vi "MT Generate MSK System Parameters.vi"(0 "samples per symbol (16)":i32=16, 5 "differential encoding enable":enum16{"disable", "enable"}(ring)=enum."enable", 11 "error in (no error)":errorcluster) -> (6 "MSK system parameters":T1, 8 "bits per symbol":i32, 15 "error out":errorcluster)   [LabVIEW 2020, in "niDMT.lvlib"]
doc: "This polymorphic instance calculates parameters for use with either the MT Modulate MSK VI or the MT Demodulate MSK VI."
uses:
  <vilib>/addons/Modulation/niDMT.lvlib
  <vilib>/addons/Modulation/Digital/Support/Controls/MSK System Parameters.ctl
  <vilib>/addons/Modulation/niAMT.lvlib
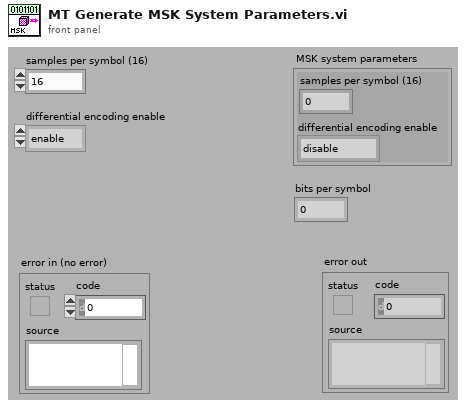
[diagram p1: front panel]
types:
  T1 = cluster{"differential encoding enable":enum16{"disable", "enable"}, "samples per symbol (16)":i32}
  T2 = typedef "niDMT.lvlib/MSK System Parameters.ctl" = cluster{"differential encoding enable":enum16{"disable", "enable"}, "samples per symbol (16)":i32}
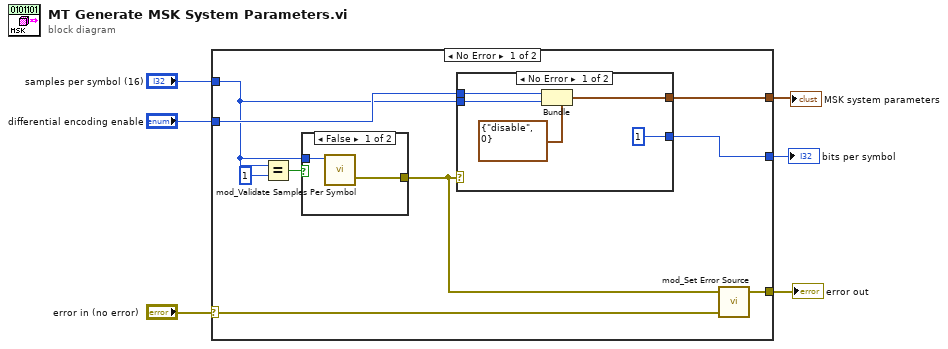
[diagram p0: block diagram]
diagram:
  n1 = case shown="No Error" "error in (no error)" {
    selector: "error in (no error)" -> [w12 w23]
    tunnel: "samples per symbol (16)" -> [w9 _]
    tunnel: [w15 _] -> w3
    tunnel: "differential encoding enable" -> [w14 _]
    tunnel: [w11 w23] -> w5
    tunnel: [w13 _] -> w1
    frame No Error {
      n2 = Equal?(x=w9, y=1) -> (x = y?=w7:bool)
      n3 = case shown="False" w7 {
        tunnel: w9 -> [w17 _]
        tunnel: [w16 _] -> w10
        frame False {
          n4 = call <vilib>:"mod_Validate Samples Per Symbol.vi"("Samples Per Symbol"=w17) -> ("error out"=w16:errorcluster)  [unwired: 10 out]
        }
        frame True {
        }
      }
      n5 = case shown="No Error" w10 {
        tunnel: [w22 _] -> w15
        tunnel: w14 -> [w21 _]
        tunnel: [1 _] -> w13
        tunnel: w9 -> [w19 _]
        frame No Error {
          n6 = Bundle(cluster=T2 {"differential encoding enable"=enum."disable", "samples per symbol (16)"=0} ("MSK system parameters"), "differential encoding enable"=w21, "samples per symbol (16)"=w19) -> (w22:T2)
        }
        frame Error {
        }
      }
      n7 = call <vilib>:"mod_Set Error Source.vi"("initial error in (no error)"=w12, "final error in (no error)"=w10) -> ("error out"=w11:errorcluster)  [unwired: 3 out]
    }
    frame Error {
    }
  }
  "MSK system parameters" <- w3
  "bits per symbol" <- w1
  "error out" <- w5
